vi "FPGA_driver.vi"() -> ()   [LabVIEW 2019]
uses:
  <vilib>/Platform/TimedLoop/XDataNode/timing_clust.ctl
  <vilib>/Platform/TimedLoop/XDataNode/nitl_modes.ctl
  <vilib>/Platform/TimedLoop/XDataNode/wakeup.ctl
  <vilib>/rvi/Emulation/niFpgaGetClockAttributes.vi
  <vilib>/rvi/Emulation/niFpgaSctlEmulationGetInTimedLoop.vi
  <vilib>/rvi/Emulation/niFpgaEmulationReportErrorSimple.vi
  <vilib>/rvi/Emulation/niFpgaProcessEmulError.vi
  <vilib>/rvi/Emulation/niFpgaCriticalErrorInLSC.vi
  <vilib>/rvi/eio/common/nirviEmuTemplateMethod_errors.vi
  <vilib>/rvi/Analysis/common/FxpNativeNode/niFpgaFxpNative.xnode
  <vilib>/eio/EIONode/EIONode.xnode
  <vilib>/platform/TimedLoop/XDataNode/XDataNode.xnode
  <vilib>/Platform/TimedLoop/XDataNode/XDNodeRunTimeDep.lvlib
panel:
  in  "ConnectorC/DIO0":bool
  out "Output Encoder 2":i32
  out "Output Encoder 1":i16
  in  "Count(mSec)":u32
  out "Encoder Position 3":i16
  in  "Num_cycle_on":u32
  in  "enable?":bool
  out "Encoder Position 2":i16
  in  "Encoder Reset 2":bool
  in  "Encoder Reload Value 2":i16
  in  "Coil Current Direction":bool
  in  "ConnectorC/AO1":i16
  in  "ConnectorC/AO0":i16
  out "ConnectorC/AI1":i16
  out "ConnectorC/AI0":i16
  out "clk/pulse":i32
  out "Velocity\nValid?":bool
  in  "Position Ref.":i32
  in  "Num Clocks\nper Period":u32=400000
  in  "Velocity \nLimit":i32=10
  in  "Position Loop\nPeriod (ms)":u32=10
  out "Encoder Position":i16
  in  "Encoder Reset":bool
  in  "Encoder Reload Value":i16
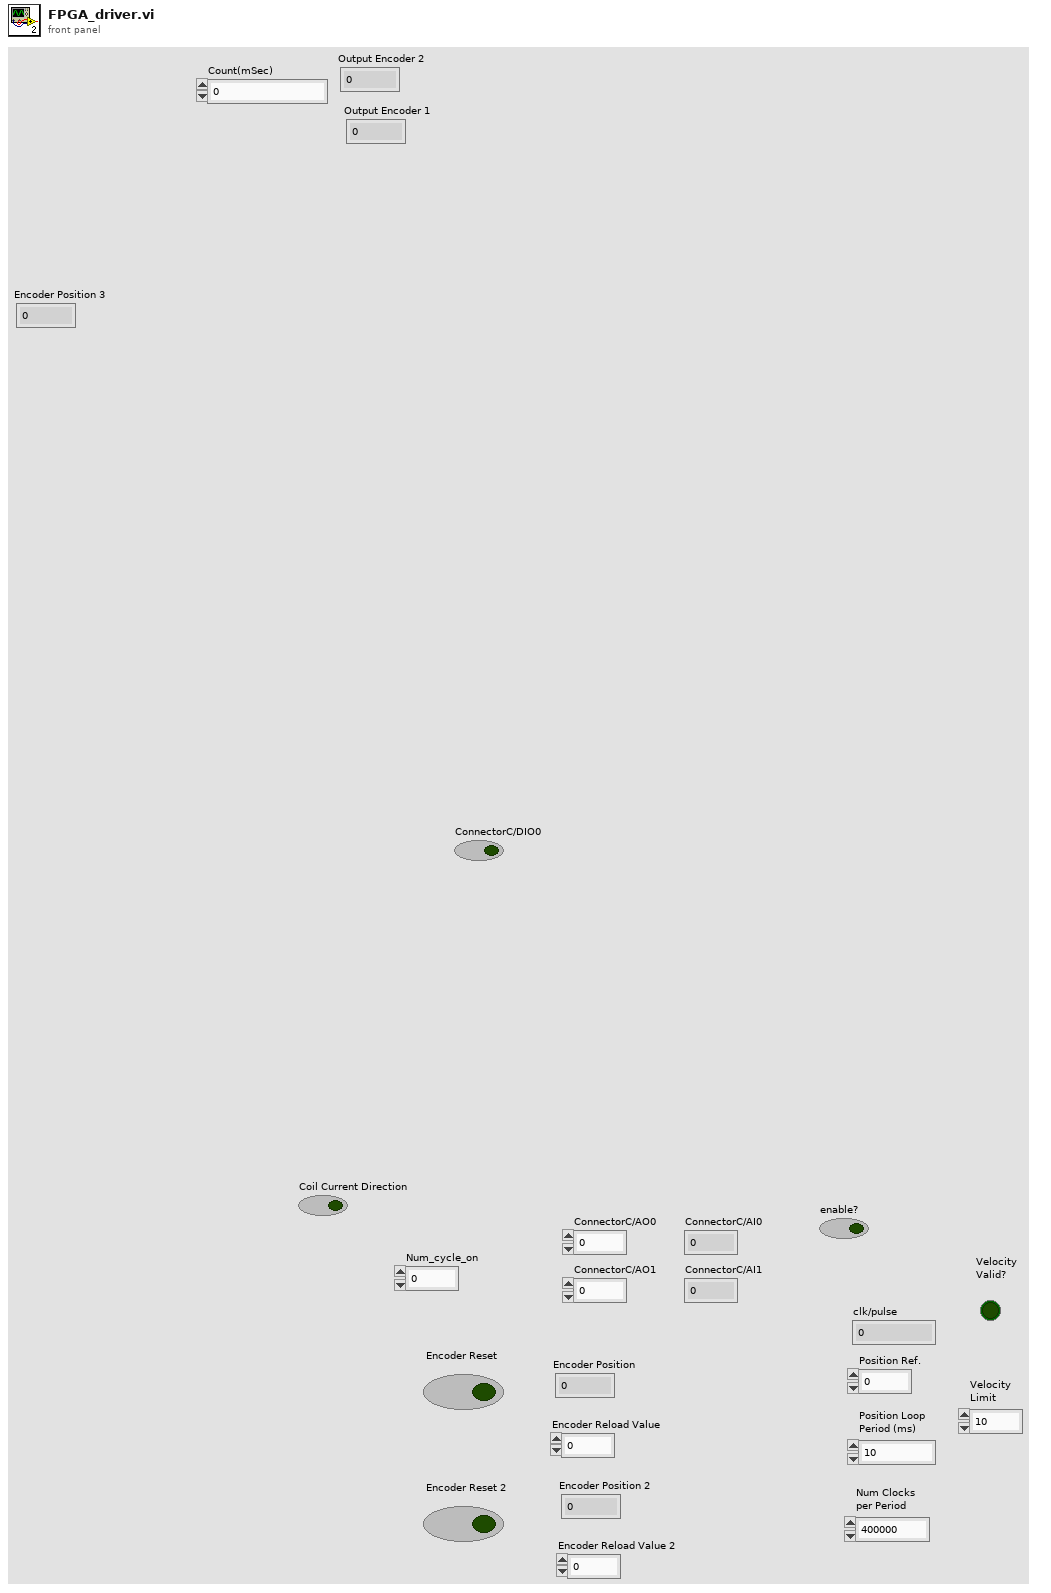
[diagram p1: front panel]
types:
  T1 = typedef "XDNodeRunTimeDep.lvlib/timing_clust.ctl" = cluster{"Expected End [f-1]":u64, "Actual End [f-1]":u64, "Finished Late? [f-1]":bool, "Expected End [i-1]":u64, "Actual End [i-1]":u64, "Finished Late? [i-1]":bool, "Expected Start [i]":u64, "Actual Start [i]":u64, "Expected Start [f]":u64, "Actual Start [f]":u64, "Source Name":string, "Structure Name":string, "Period":i64, "Deadline":i64, "Offset":i64, "Start":i64, "Priority":i32, "Timeout":i32, "Mode":T2, "Wakeup Reason":T3, "Error":errorcluster, "Source Type":string, "Secondary Source Type":string, "Global End Time":u64, "Global Start Time":u64, "Frame Duration":u64, "Iteration Duration":u64, "Assigned CPU":i32, "I/O Scan Engine Mode":u32}
  T2 = typedef "XDNodeRunTimeDep.lvlib/nitl_modes.ctl" = enum32{"No Change", "Process missed periods, maintain original phase", "Discard missed periods, maintain original phase", "Process missed periods, ignore original phase", "Discard missed periods, ignore original phase"}
  T3 = typedef "XDNodeRunTimeDep.lvlib/wakeup.ctl" = enum32{"Normal", "Aborted", "Asynchronous wakeup", "Timing source error", "Timed loop error", "Timeout"}
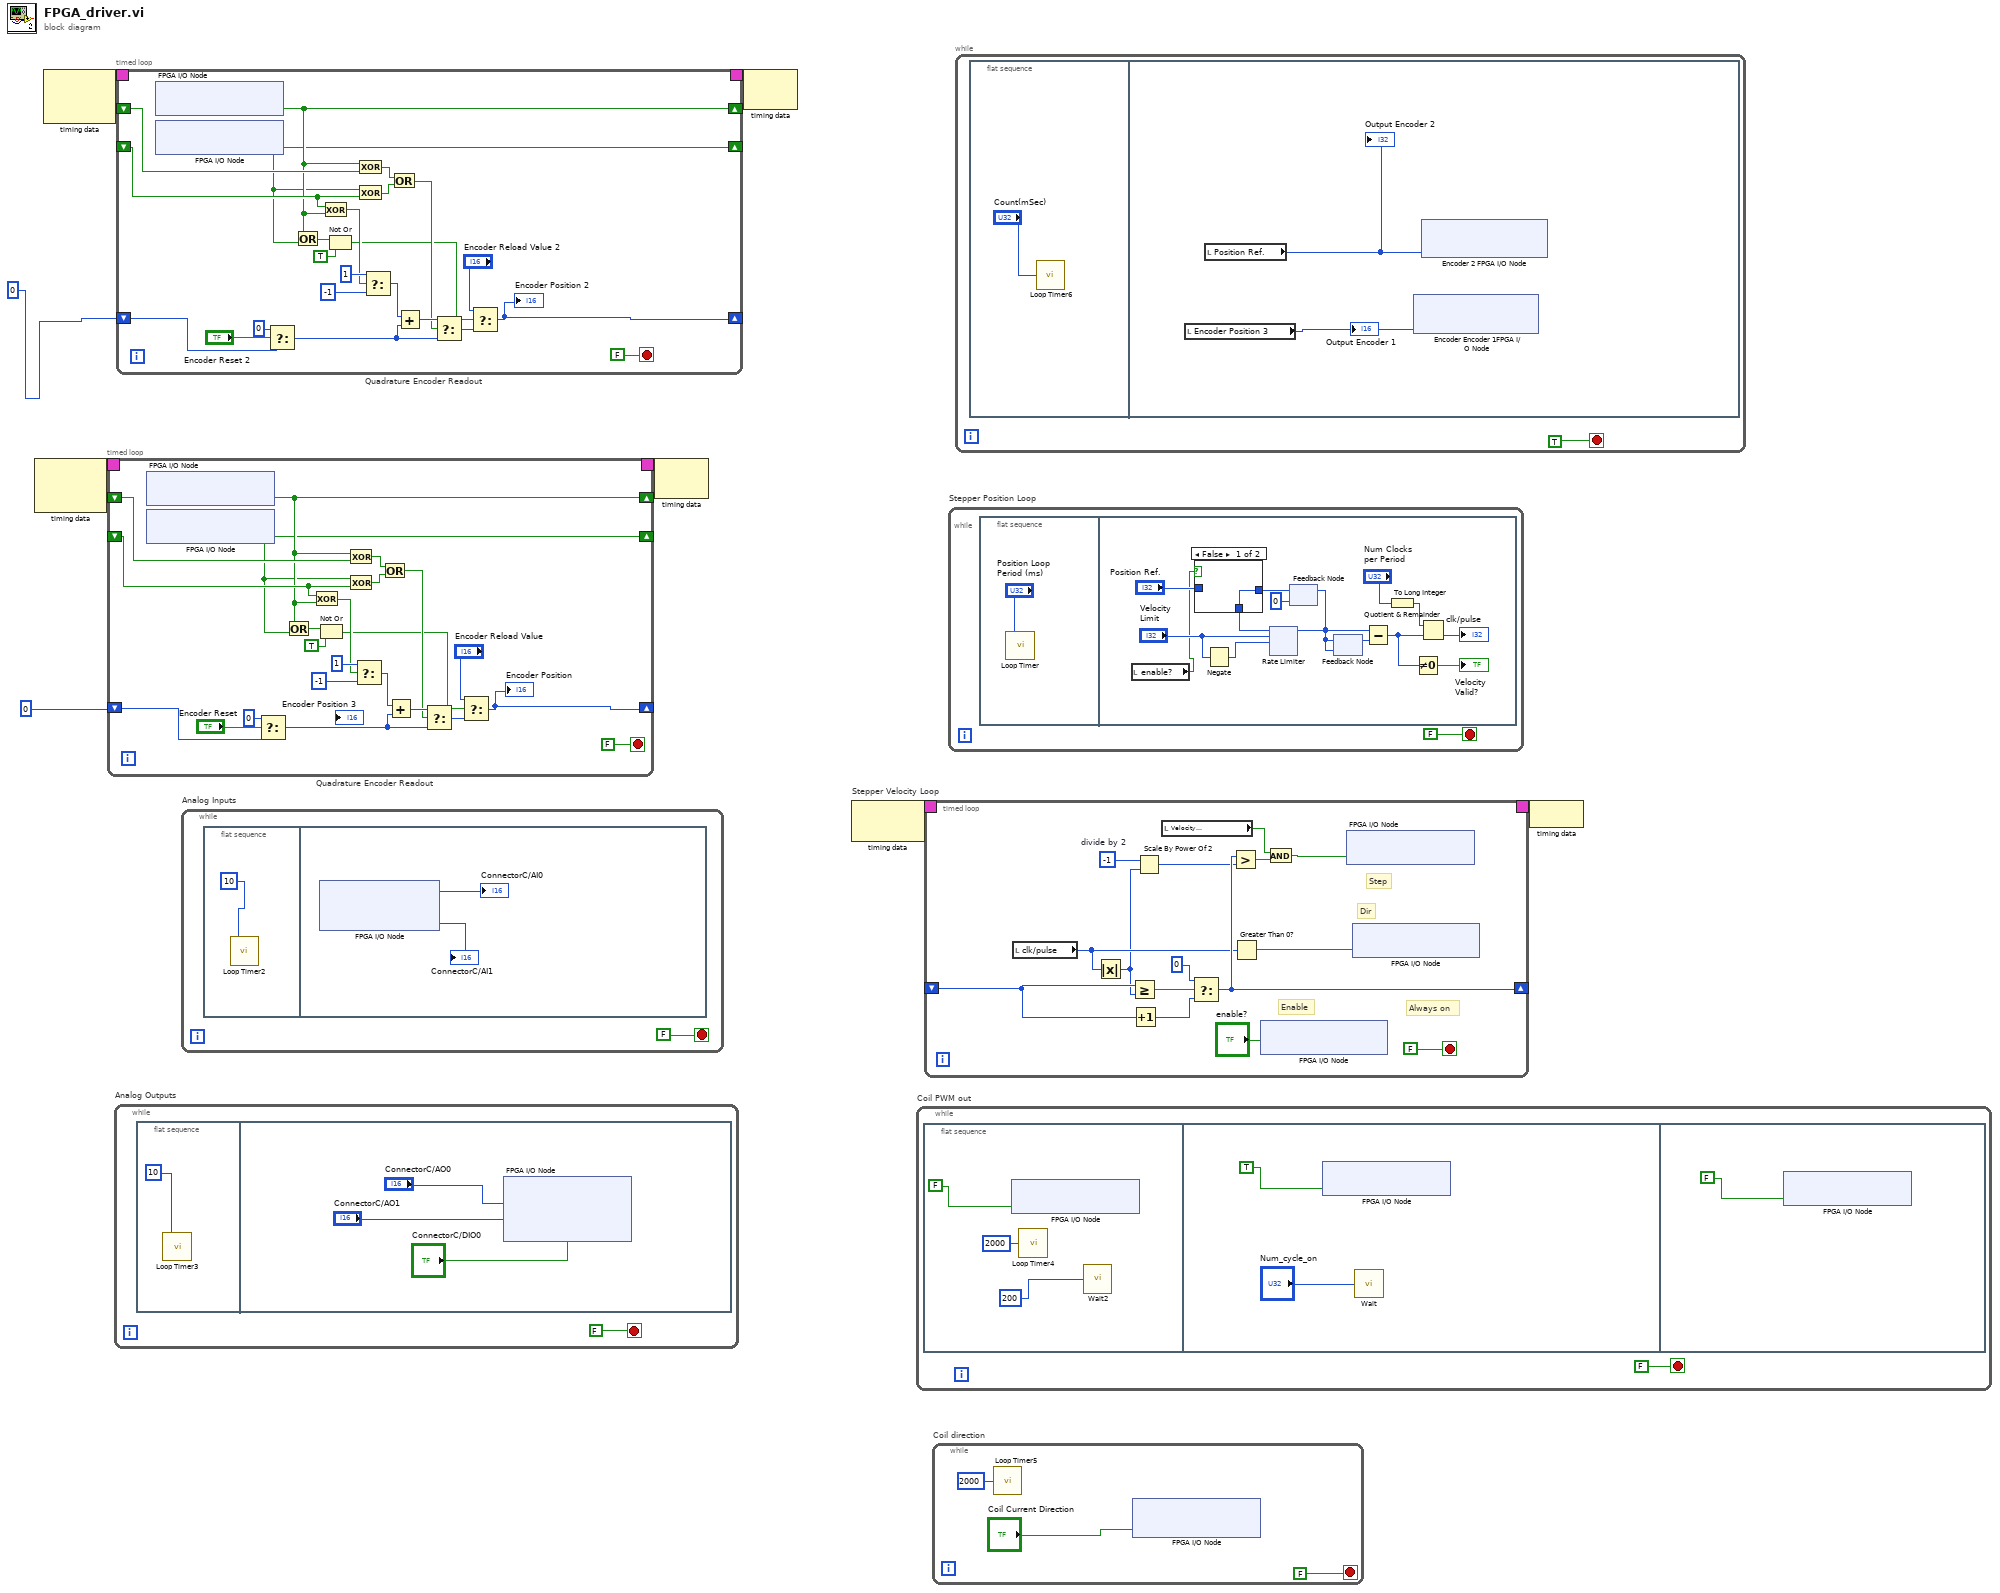
[diagram p0: block diagram]
diagram:
  n1 = node-c288() -> (w8:T1)  [unwired: 2 out]
  n2 = node-c288() -> (w3:T1)  [unwired: 2 out]
  n3 = timed-loop "Quadrature Encoder Readout" {
    timing-out: [_] -> w7
    timing: w8 -> [_]
    shift-left: _ -> [w16]
    shift-right: [w9] -> _
    shift-left: i16 0 -> [w27]
    shift-right: [w10] -> _
    shift-left: _ -> [w17]
    shift-right: [w13] -> _
    stop <- FALSE stop-if-true
    n4 = xnode "FPGA I/O Node"() -> ("ConnectorA/DIO0"=w13:bool)  [unwired: 1 in, 1 out]
    n5 = xnode "FPGA I/O Node"() -> ("ConnectorA/DIO1"=w9:bool)  [unwired: 1 in, 1 out]
    n6 = Select(t=i16 0, s="Encoder Reset", f=w27) -> (s? t:f=w29:i16)
    n7 = Or(x=w13, y=w9) -> (x .or. y?=w12:bool)
    n8 = Exclusive Or(1:w13, 2:w16) -> (0:w18:bool)
    n9 = Not Or(1:TRUE ("y"), 2:w12) -> (0:w15:bool)
    n10 = Exclusive Or(1:w17, 2:w13) -> (0:w20:bool)
    n11 = Exclusive Or(1:w16, 2:w9) -> (0:w21:bool)
    n12 = Select(t=i16 1, s=w18, f=i16 -1) -> (s? t:f=w26:i16)
    n13 = Or(x=w20, y=w21) -> (x .or. y?=w19:bool)
    n14 = Add(x=w26, y=w29) -> (x+y=w31:i16)
    n15 = Select(t=w31, s=w19, f=w29) -> (s? t:f=w23:i16)
    n16 = Select(t="Encoder Reload Value", s=w15, f=w23) -> (s? t:f=w10:i16)
    "Encoder Position" <- w10
  }
  n17 = while "Analog Outputs" {
    stop <- FALSE stop-if-true
    n18 = flat-sequence {
      frame #0 {
        n19 = call "Loop Timer3"("Count(uSec)"=u32 10) -> ()  [unwired: 1 out]
      }
      frame #1 {
        n20 = xnode "FPGA I/O Node"("ConnectorC/AO0"="ConnectorC/AO0", "ConnectorC/AO1"="ConnectorC/AO1", "ConnectorC/DIO0"="ConnectorC/DIO0") -> ()  [unwired: 3 in, 3 out]
      }
    }
  }
  n21 = timed-loop "Quadrature Encoder Readout" {
    timing-out: [_] -> w2
    timing: w3 -> [_]
    shift-left: _ -> [w46]
    shift-right: [w39] -> _
    shift-left: i16 0 -> [w57]
    shift-right: [w40] -> _
    shift-left: _ -> [w47]
    shift-right: [w43] -> _
    stop <- FALSE stop-if-true
    n22 = xnode "FPGA I/O Node"() -> ("ConnectorA/DIO2"=w43:bool)  [unwired: 1 in, 1 out]
    n23 = xnode "FPGA I/O Node"() -> ("ConnectorA/DIO3"=w39:bool)  [unwired: 1 in, 1 out]
    n24 = Select(t=i16 0, s="Encoder Reset 2", f=w57) -> (s? t:f=w59:i16)
    n25 = Or(x=w43, y=w39) -> (x .or. y?=w42:bool)
    n26 = Exclusive Or(1:w43, 2:w46) -> (0:w48:bool)
    n27 = Not Or(1:TRUE ("y"), 2:w42) -> (0:w45:bool)
    n28 = Exclusive Or(1:w47, 2:w43) -> (0:w50:bool)
    n29 = Exclusive Or(1:w46, 2:w39) -> (0:w51:bool)
    n30 = Select(t=i16 1, s=w48, f=i16 -1) -> (s? t:f=w56:i16)
    n31 = Or(x=w50, y=w51) -> (x .or. y?=w49:bool)
    n32 = Add(x=w56, y=w59) -> (x+y=w61:i16)
    n33 = Select(t=w61, s=w49, f=w59) -> (s? t:f=w53:i16)
    n34 = Select(t="Encoder Reload Value 2", s=w45, f=w53) -> (s? t:f=w40:i16)
    "Encoder Position 2" <- w40
  }
  n35 = while "Analog Inputs" {
    stop <- FALSE stop-if-true
    n36 = flat-sequence {
      frame #0 {
        n37 = call "Loop Timer2"("Count(uSec)"=u32 10) -> ()  [unwired: 1 out]
      }
      frame #1 {
        n38 = xnode "FPGA I/O Node"() -> ("ConnectorC/AI0"=→"ConnectorC/AI0":i16, "ConnectorC/AI1"=→"ConnectorC/AI1":i16)  [unwired: 2 in, 2 out]
      }
    }
  }
  n39 = node-c288(w7) -> ()  [unwired: 1 out]
  n40 = node-c288(w2) -> ()  [unwired: 1 out]
  n41 = node-c288() -> (w5:T1)  [unwired: 1 in]
  n42 = while "Coil PWM out" {
    stop <- FALSE stop-if-true
    n43 = flat-sequence {
      frame #0 {
        n44 = xnode "FPGA I/O Node"("ConnectorC/DIO1"=FALSE) -> ()  [unwired: 1 in, 1 out]
        n45 = call "Loop Timer4"("Count(Ticks)"=u32 2000 ("Count(uSec)")) -> ()  [unwired: 1 out]
        n46 = call "Wait2"("Count(Ticks)"=u32 200) -> ()  [unwired: 1 out]
      }
      frame #1 {
        n47 = xnode "FPGA I/O Node"("ConnectorC/DIO1"=TRUE) -> ()  [unwired: 1 in, 1 out]
        n48 = call "Wait"("Count(Ticks)"="Num_cycle_on") -> ()  [unwired: 1 out]
      }
      frame #2 {
        n49 = xnode "FPGA I/O Node"("ConnectorC/DIO1"=FALSE) -> ()  [unwired: 1 in, 1 out]
      }
    }
  }
  n50 = timed-loop "Stepper Velocity Loop" {
    timing: w5 -> [_]
    timing-out: [_] -> w4
    shift-right: [w85] -> _
    shift-left: _ -> [w82]
    stop <- FALSE stop-if-true
    w78 = -1  # divide by 2
    # "Always on"
    # "Enable"
    # "Dir"
    # "Step"
    n51 = local read "clk/pulse"() -> (w81:i32)
    n52 = Absolute Value(x=w81) -> (abs(x)=w79:i32)
    n53 = Greater Or Equal?(x=w82, y=w79) -> (x >= y?=w86:bool)
    n54 = Increment(x=w82) -> (x+1=w88:i32)
    n55 = Scale By Power Of 2(n=w78, x=w79) -> (x*2^n=w80:i32)
    n56 = local read "Velocity\nValid?"() -> (w83:bool)
    n57 = Select(t=0, s=w86, f=w88) -> (s? t:f=w85:i32)
    n58 = Greater?(x=w85, y=w80) -> (0:w84:bool)
    n59 = Greater Than 0?(x=w81) -> (x > 0?=w77:bool)
    n60 = xnode "FPGA I/O Node"("ConnectorC/DIO4"="enable?") -> ()  [unwired: 1 in, 1 out]
    n61 = And(x=w83, y=w84) -> (x .and. y?=w76:bool)
    n62 = xnode "FPGA I/O Node"("ConnectorC/DIO2"=w76) -> ()  [unwired: 1 in, 1 out]
    n63 = xnode "FPGA I/O Node"("ConnectorC/DIO3"=w77) -> ()  [unwired: 1 in, 1 out]
  }
  n64 = while "Coil direction" {
    stop <- FALSE stop-if-true
    n65 = call "Loop Timer5"("Count(Ticks)"=u32 2000 ("Count(uSec)")) -> ()  [unwired: 1 out]
    n66 = xnode "FPGA I/O Node"("ConnectorC/DIO0"="Coil Current Direction") -> ()  [unwired: 2 in, 2 out]
  }
  n67 = while "Stepper Position Loop" {
    stop <- FALSE stop-if-true
    n68 = flat-sequence {
      frame #0 {
        n69 = call "Loop Timer"("Count(mSec)"="Position Loop\nPeriod (ms)") -> ()  [unwired: 1 out]
      }
      frame #1 {
        n70 = local read "enable?"() -> (w97:bool)
        n71 = Negate(x="Velocity \nLimit") -> (-x=w104:i32)
        n72 = feedback #1(0 ("output")) -> (w99:i32)
        n73 = case shown="False" w97 {
          tunnel: [w111 w112] -> w102
          tunnel: "Position Ref." -> [_ w112]
          tunnel: w99 -> [w111 _]
          frame False {
          }
          frame True {
          }
        }
        n74 = xnode ("Rate Limiter")("pos slew rate * dt"="Velocity \nLimit", "input"=w102, "neg slew rate * dt"=w104) -> ("output"=w100:i32)  [unwired: 1 in]
        n75 = feedback-in #1(w100) -> ()
        n76 = feedback #2(w100) -> (w109:i32)
        n77 = feedback-in #2(w100) -> ()
        n78 = Subtract(x=w100, y=w109) -> (x-y=w106:i32)
        n79 = To Long Integer(number="Num Clocks\nper Period") -> (32bit integer=w107:i32)
        n80 = Not Equal To 0?(x=w106) -> (x != 0?=→"Velocity\nValid?":bool)
        n81 = Quotient & Remainder(x=w107, y=w106) -> (floor(x/y)=→"clk/pulse":i32)  [unwired: 1 out]
      }
    }
  }
  n82 = while {
    stop <- TRUE stop-if-true
    n83 = flat-sequence {
      frame #0 {
        n84 = call "Loop Timer6"("Count(mSec)"="Count(mSec)") -> ()  [unwired: 1 out]
      }
      frame #1 {
        n85 = local read "Encoder Position 3"() -> (w139:i16)
        "Output Encoder 1" <- w139
        n86 = local read "Position Ref."() -> (w140:i32)
        "Output Encoder 2" <- w140
        n87 = xnode "Encoder Encoder 1FPGA I/O Node"("ConnectorC/AO1"=w139) -> ()  [unwired: 2 in, 2 out]
        n88 = xnode "Encoder 2 FPGA I/O Node"("ConnectorC/AO0"=w140) -> ()  [unwired: 2 in, 2 out]
      }
    }
  }
  n89 = node-c288(w4) -> ()
